vi "Init Module.vi"(8 "error in":errorcluster, 11 "Singleton Module Admin in":refnum<class "Delacor_lib_QMH_Module Admin.lvclass">) -> (0 "error out":errorcluster, 2 "Scripting Server Request Events":T1, 3 "Singleton Module Admin out":refnum<class "Delacor_lib_QMH_Module Admin.lvclass">)   [LabVIEW 2025, in "Scripting Server.lvlib"]
doc: "Initialize the module by creating Broadcast Events, Request Events, and synchronization rendezvous.\n_____\nBased on DQMH Dev Tools: Project Template 7.1.0.1503."
uses:
  Scripting Server.lvlib
  <vilib>/Delacor/Delacor QMH/Libraries/Module Admin_class/Delacor_lib_QMH_Module Admin.lvclass
  Request Events--cluster.ctl
  Stop Argument--cluster.ctl
  Show Panel Argument--cluster.ctl
  Hide Panel Argument--cluster.ctl
  Get Module Execution Status Argument--cluster.ctl
  Show Diagram Argument--cluster.ctl
  New VI Argument--cluster.ctl
  New VI (Reply Payload)--cluster.ctl
  Add Object Argument--cluster.ctl
  Add Object (Reply Payload)--cluster.ctl
  Connect Objects Argument--cluster.ctl
  Connect Objects (Reply Payload)--cluster.ctl
  Get Object Terminals Argument--cluster.ctl
  Get Object Terminals (Reply Payload)--cluster.ctl
  get vi error list Argument--cluster.ctl
  get vi error list (Reply Payload)--cluster.ctl
  Cleanup VI Argument--cluster.ctl
  Cleanup VI (Reply Payload)--cluster.ctl
  create_control Argument--cluster.ctl
  create_control (Reply Payload)--cluster.ctl
  Run VI Argument--cluster.ctl
  Run VI (Reply Payload)--cluster.ctl
  add_to_selection Argument--cluster.ctl
  add_to_selection (Reply Payload)--cluster.ctl
  clear_selection_list Argument--cluster.ctl
  clear_selection_list (Reply Payload)--cluster.ctl
  remove_from_selection Argument--cluster.ctl
  remove_from_selection (Reply Payload)--cluster.ctl
  enclose_selection Argument--cluster.ctl
  enclose_selection (Reply Payload)--cluster.ctl
  rename_object Argument--cluster.ctl
  rename_object (Reply Payload)--cluster.ctl
  set_value Argument--cluster.ctl
  set_value (Reply Payload)--cluster.ctl
  delete_object Argument--cluster.ctl
  delete_object (Reply Payload)--cluster.ctl
  save_vi Argument--cluster.ctl
  save_vi (Reply Payload)--cluster.ctl
  get_structure_diagram Argument--cluster.ctl
  get_structure_diagram (Reply Payload)--cluster.ctl
  add_subvi Argument--cluster.ctl
  add_subvi (Reply Payload)--cluster.ctl
  connect_to_pane Argument--cluster.ctl
  connect_to_pane (Reply Payload)--cluster.ctl
  get_object_help Argument--cluster.ctl
  get_object_help (Reply Payload)--cluster.ctl
  get_loop_conditional_terminal Argument--cluster.ctl
  get_loop_conditional_terminal (Reply Payload)--cluster.ctl
  show_conditional_terminal Argument--cluster.ctl
  show_conditional_terminal (Reply Payload)--cluster.ctl
  get_loop_iteration_terminal Argument--cluster.ctl
  get_loop_iteration_terminal (Reply Payload)--cluster.ctl
  Read Config Data Argument--cluster.ctl
  get_allowed_paths Argument--cluster.ctl
  get_allowed_paths (Reply Payload)--cluster.ctl
  create_project Argument--cluster.ctl
  create_project (Reply Payload)--cluster.ctl
  Set Allowed Paths Argument--cluster.ctl
  open_vi Argument--cluster.ctl
  open_vi (Reply Payload)--cluster.ctl
  Register MCP Events Argument--cluster.ctl
  <vilib>/jgoebel/LabVIEW MCP Server SDK/MCP Server.lvlibp/Praesentationen/MCP in LabVIEW/LabVIEW-MCP-Server-Toolkit/src/MCP Server/User Events.ctl
  <vilib>/jgoebel/LabVIEW MCP Server SDK/MCP Server.lvlibp/Praesentationen/MCP in LabVIEW/LabVIEW-MCP-Server-Toolkit/src/MCP Server/onLog.ctl
  <vilib>/jgoebel/LabVIEW MCP Server SDK/MCP Server.lvlibp/Praesentationen/MCP in LabVIEW/LabVIEW-MCP-Server-Toolkit/src/MCP Server/onConnect.ctl
  <vilib>/jgoebel/LabVIEW MCP Server SDK/MCP Server.lvlibp/Praesentationen/MCP in LabVIEW/LabVIEW-MCP-Server-Toolkit/src/MCP Server/onToolsList.ctl
  <vilib>/jgoebel/LabVIEW MCP Server SDK/MCP Server.lvlibp/Praesentationen/MCP in LabVIEW/LabVIEW-MCP-Server-Toolkit/src/MCP Server/onToolsCall.ctl
  <vilib>/jgoebel/LabVIEW MCP Server SDK/MCP Server.lvlibp/Praesentationen/MCP in LabVIEW/LabVIEW-MCP-Server-Toolkit/src/MCP Server/onNotification.ctl
  <vilib>/jgoebel/LabVIEW MCP Server SDK/MCP Server.lvlibp/Praesentationen/MCP in LabVIEW/LabVIEW-MCP-Server-Toolkit/src/MCP Server/onTool.ctl
  <vilib>/jgoebel/LabVIEW MCP Server SDK/MCP Server.lvlibp/Praesentationen/MCP in LabVIEW/LabVIEW-MCP-Server-Toolkit/src/MCP Server/Tool Data.ctl
  <vilib>/jgoebel/LabVIEW MCP Server SDK/MCP Server.lvlibp/Praesentationen/MCP in LabVIEW/LabVIEW-MCP-Server-Toolkit/src/MCP Server/Input Parameter.ctl
  <vilib>/jgoebel/LabVIEW MCP Server SDK/MCP Server.lvlibp/Praesentationen/MCP in LabVIEW/LabVIEW-MCP-Server-Toolkit/src/MCP Server/Output Parameter.ctl
  <vilib>/jgoebel/LabVIEW MCP Server SDK/MCP Server.lvlibp/Praesentationen/MCP in LabVIEW/LabVIEW-MCP-Server-Toolkit/src/MCP Server/onRpc.ctl
  New MCP RPC Message Argument--cluster.ctl
  <vilib>/jgoebel/LabVIEW MCP Server SDK/MCP Server.lvlibp
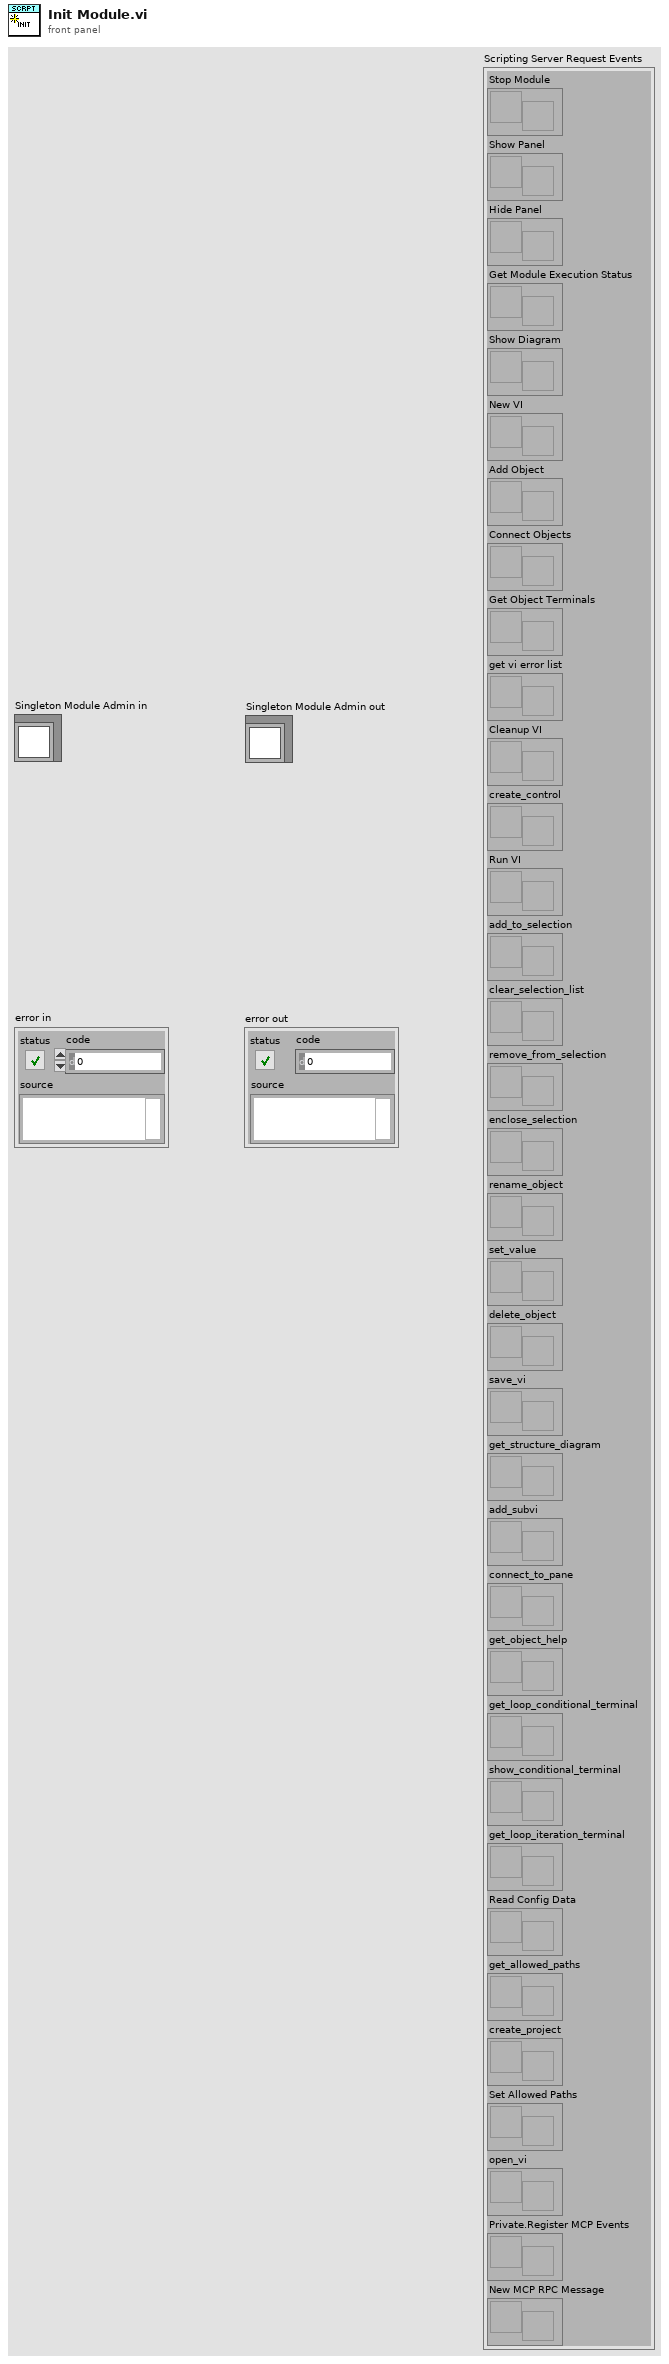
[diagram p1: front panel]
types:
  T1 = typedef "Scripting Server.lvlib/Request Events--cluster.ctl" = cluster{"Stop Module":refnum<user-event>, "Show Panel":refnum<user-event>, "Hide Panel":refnum<user-event>, "Get Module Execution Status":refnum<user-event>, "Show Diagram":refnum<user-event>, "New VI":refnum<user-event>, "Add Object":refnum<user-event>, "Connect Objects":refnum<user-event>, "Get Object Terminals":refnum<user-event>, "get vi error list":refnum<user-event>, "Cleanup VI":refnum<user-event>, "create_control":refnum<user-event>, "Run VI":refnum<user-event>, "add_to_selection":refnum<user-event>, "clear_selection_list":refnum<user-event>, "remove_from_selection":refnum<user-event>, "enclose_selection":refnum<user-event>, "rename_object":refnum<user-event>, "set_value":refnum<user-event>, "delete_object":refnum<user-event>, "save_vi":refnum<user-event>, "get_structure_diagram":refnum<user-event>, "add_subvi":refnum<user-event>, "connect_to_pane":refnum<user-event>, "get_object_help":refnum<user-event>, "get_loop_conditional_terminal":refnum<user-event>, "show_conditional_terminal":refnum<user-event>, "get_loop_iteration_terminal":refnum<user-event>, "Read Config Data":refnum<user-event>, "get_allowed_paths":refnum<user-event>, "create_project":refnum<user-event>, "Set Allowed Paths":refnum<user-event>, "open_vi":refnum<user-event>, "Private.Register MCP Events":refnum<user-event>, "New MCP RPC Message":refnum<user-event>}
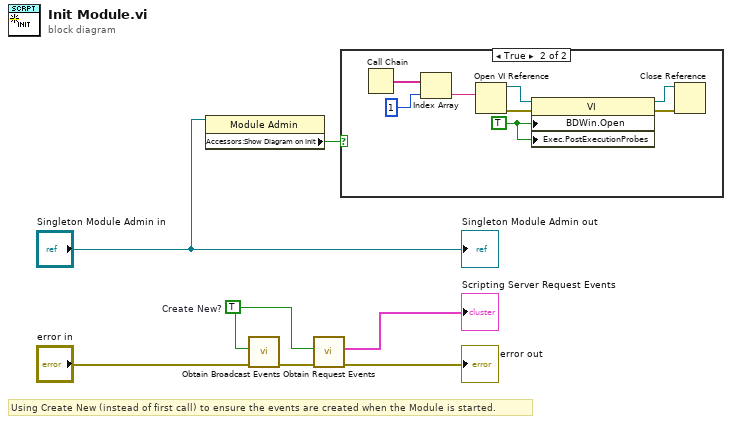
[diagram p0: block diagram]
diagram:
  w4 = TRUE  # Create New?
  # "Using Create New (instead of first call) to ensure the events are created when the Module is started."
  n1 = property class="Module Admin"(reference="Singleton Module Admin in") -> ("Accessors:Show Diagram on Init"=w2:bool)  [unwired: 1 in, 2 out]
  n2 = call "Obtain Broadcast Events.vi"("error in"="error in", "Create New? (F)"=w4) -> ("error out"=w7:errorcluster)  [unwired: 8 in, 1 out]
  n3 = call "Obtain Request Events.vi"("error in"=w7, "Create New? (F)"=w4) -> ("error out"=→"error out":errorcluster, "Scripting Server Request Events"=→"Scripting Server Request Events":T1)  [unwired: 8 in]
  n4 = case shown="True" w2 {
    frame False {
    }
    frame True {
      w11 = TRUE ("Block Diagram Window:Open")
      n5 = Call Chain() -> (call chain=w15:string[])
      n6 = Index Array(array=w15, index=1) -> (element=w8:string)
      n7 = Open VI Reference(vi path=w8) -> (vi reference=w12:refnum<vi>, error out=w13:errorcluster)  [unwired: 5 in]
      n8 = property class="VI"(reference=w12, error in=w13, "BDWin.Open"=w11, "Exec.PostExecutionProbes"=w11) -> (reference out=w9:refnum<vi>, error out=w10:errorcluster)
      n9 = Close Reference(reference=w9, error in (no error)=w10) -> ()  [unwired: 1 out]
    }
  }
  "Singleton Module Admin out" <- "Singleton Module Admin in"
